vi "ADC_wave_sample.vi"() -> ()   [LabVIEW 2022 SP3]
uses:
  libdaqVI.lvlib
panel:
  in  "量程选择":T1(ring)=enum."0-5V"
  in  "AIN7":bool=TRUE
  in  "AIN5":bool=TRUE
  in  "AIN6":bool=TRUE
  in  "AIN4":bool=TRUE
  in  "AIN3":bool=TRUE
  in  "AIN2":bool=TRUE
  in  "AIN1":bool=TRUE
  in  "AIN0":bool=TRUE
  in  "wave_len":i32=1000 caption="波形显示长度"
  out "Total_len":i32 caption="每通道累计采集数据长度"
  in  "停止采集":bool
  in  "开始采集":bool
  out "设备名称":string
  in  "采样模式":enum16{"序列采样", "分组采样", "同步采样"}(ring)
  in  "组间隔(us)":u32=1000
  in  "采样次数":u32
  in  "采样频率(Hz)":u32=10000 format="%.0p"
  out "采集卡状态":bool
  out "设备数量":u32
  out "波形图":dbl[][](graph)
  in  "退出程序":bool
  # "范例说明：\n1、范例支持的采集卡：DAQ-USB3212、DAQ-USB3213、DAQ-USB3214\n2、参数配置\n1）量程选择：\nDAQ-USB3212 支持量程:0-5V\nDAQ-USB3213 支持量程:0-2.5V/0-5V/0-10V\nDAQ-USB3214 支持量程:0-2.5V/0-5V/0-10V/±2.5V/±5V/±10V\n必须选择正确的量程，否则程序会报错\n2）采样频率最大支持100kHz，同步采样时，8通道最大为10KHz\n3）采样次数，0代表无限次采样，非0值代表每通道的采样点个数\n各种采样模式之间的区别，以及详细的使用方法，请参考API手册\n3、配置正确参数之后，再开始运行程序，程序运行之后将无法修改参数\n4、程序运行之后，点击“开始采集”，进行数据采集，停止采集之后点击“开始采集”可以再次开启采集过程；"
  # "DAQ-ADC1波形采样演示程序"
  # "通道选择"
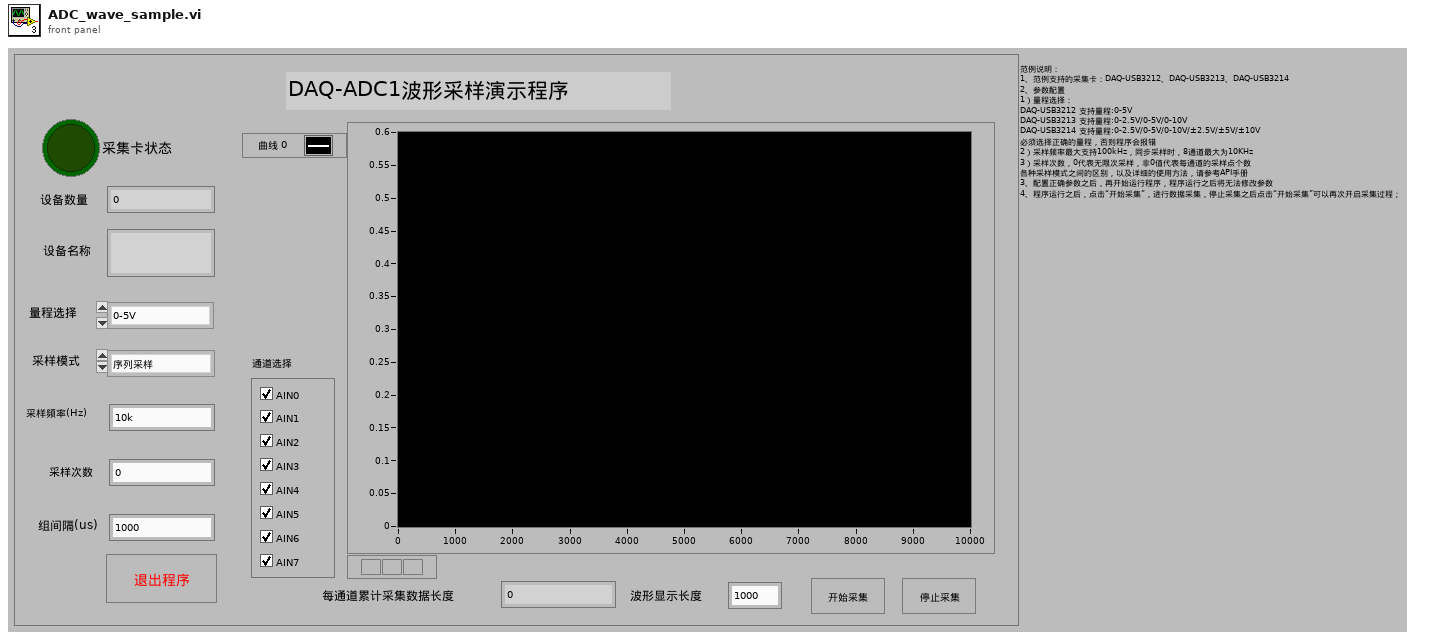
[diagram p1: front panel]
types:
  T1 = enum16{"0-1V", "0-2V", "0-2.5V", "0-5V", "0-10V", "±78.125mV", "±156.25mV", "±312.5mV", "±0.256V", "±0.512V", "±0.625V", "±1V", "±1.024V", "±1.25V", "±2V", "±2.048V", "±2.5V", "±4.096V", "±5.0V", "±10V", "0-20mA", "±20mA", "0-40mA", "±40mA"}
  T2 = cluster{"channel_list ":u8[], "channel_count":u8, "sample_mode":u8, "frequency":u32, "cycles":u32, "group_interval":u32}
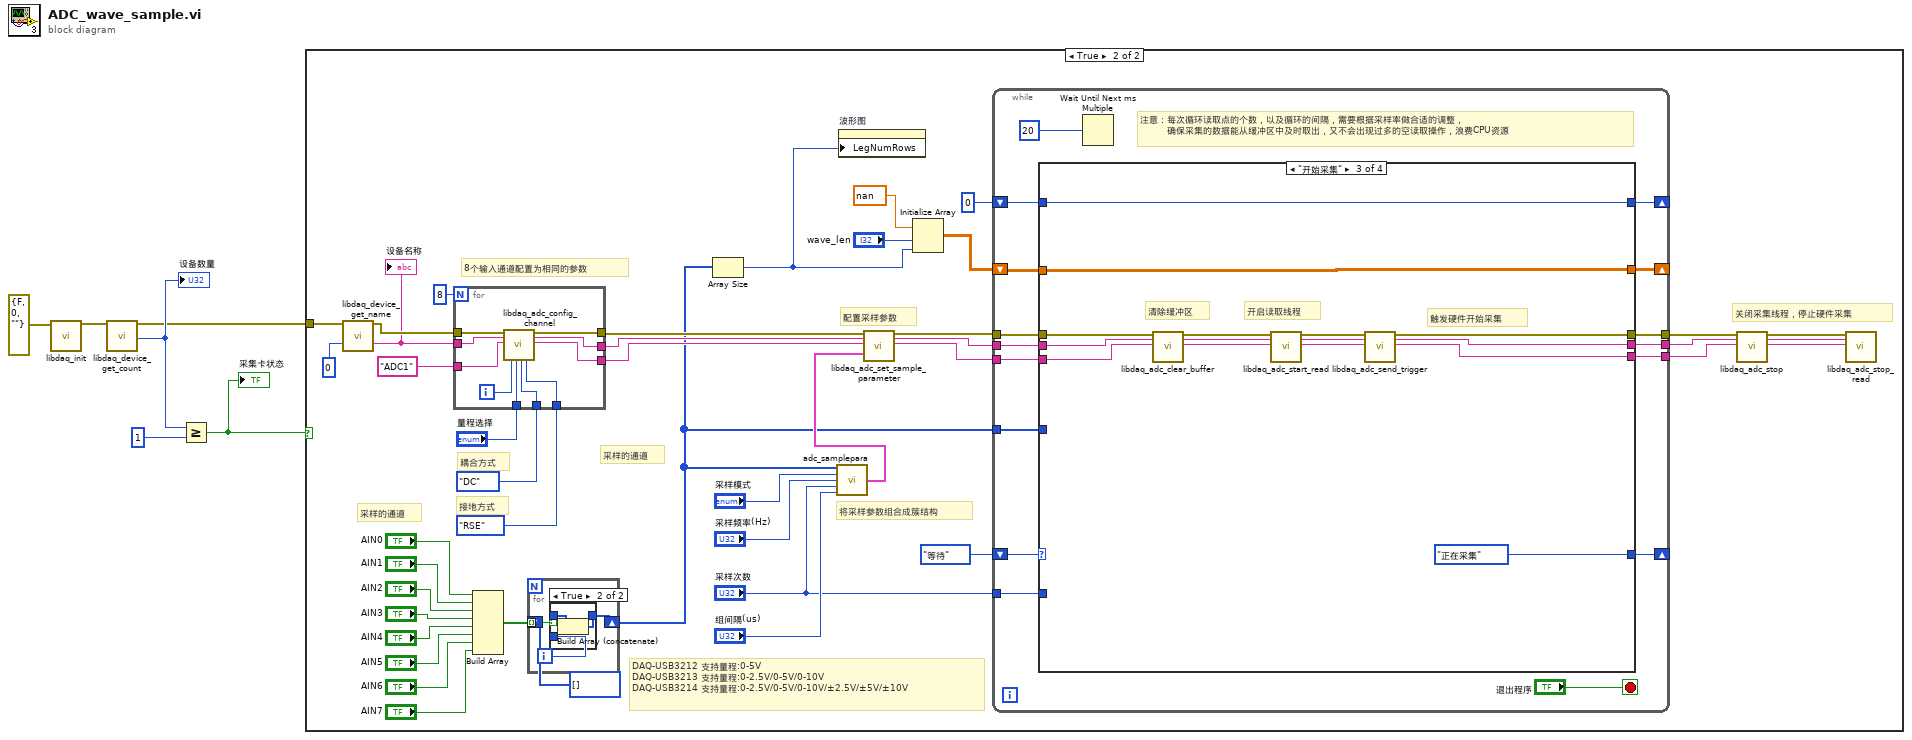
[diagram p0: block diagram]
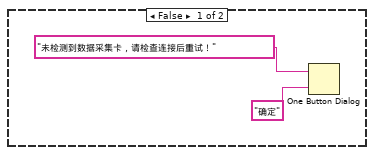
[diagram p2: hidden frame]
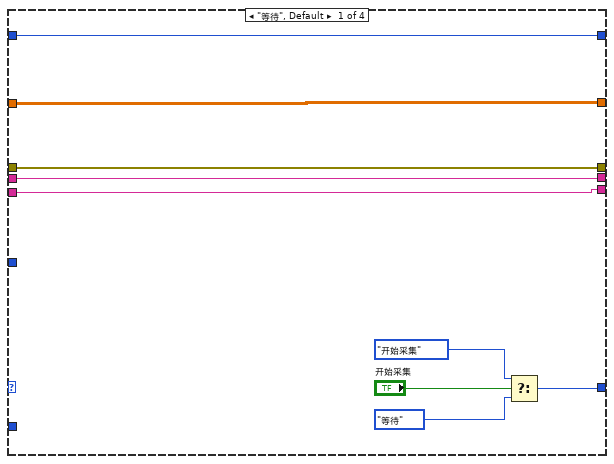
[diagram p4: hidden frame]
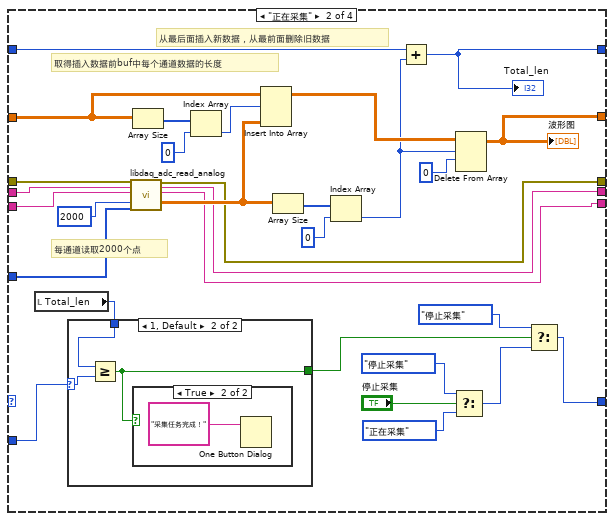
[diagram p5: hidden frame]
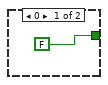
[diagram p6: hidden frame]
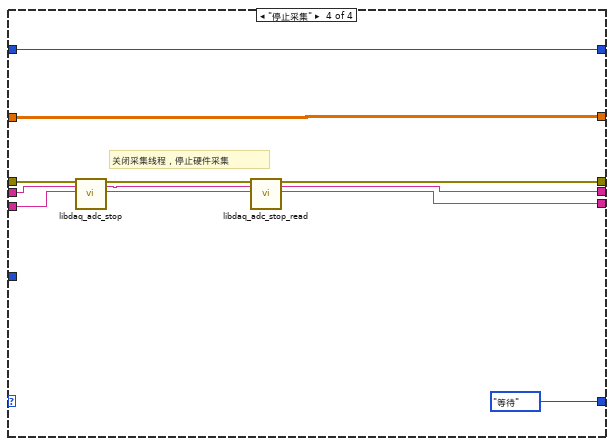
[diagram p8: hidden frame]
diagram:
  n1 = call "libdaq_init.vi"("error in (no error)"=errorcluster {"status"=FALSE, "code"=0, "source"=""}) -> ("error out"=w4:errorcluster)  [unwired: 18 in]
  n2 = call "libdaq_device_get_count.vi"("error in (no error)"=w4) -> ("error out"=w1:errorcluster, "device_count"=w2:i32)  [unwired: 17 in]
  "设备数量" <- w2
  n3 = Greater Or Equal?(x=w2, y=u32 1 ("name length")) -> (x >= y?=w3:bool)
  "采集卡状态" <- w3
  n4 = case shown="True" w3 {
    tunnel: w1 -> [_ w51]
    frame False {
      n5 = One Button Dialog(message="未检测到数据采集卡，请检查连接后重试！" ("消息"), button name ("OK")="确定" ("按钮名称（“确定”）")) -> ()  [unwired: 1 out]
    }
    frame True {
      # "关闭采集线程，停止硬件采集"
      # "采样的通道"
      # "DAQ-USB3212 支持量程:0-5V\nDAQ-USB3213 支持量程:0-2.5V/0-5V/0-10V\nDAQ-USB3214 支持量程:0-2.5V/0-5V/0-10V/±2.5V/±5V/±10V"
      # "采样的通道"
      # "接地方式"
      # "耦合方式"
      # "将采样参数组合成簇结构"
      # "配置采样参数"
      # "8个输入通道配置为相同的参数"
      n6 = call "libdaq_device_get_name.vi"("error in (no error)"=w51, "device_index"=u32 0 ("name length")) -> ("error out"=w50:errorcluster, "device_name"=w38:string)  [unwired: 16 in]
      "设备名称" <- w38
      n7 = for {
        N: 8 -> [_]
        tunnel: w50 -> [w69]
        tunnel: [w68] -> w46
        tunnel: [w64] -> w42
        tunnel: [w63] -> w41
        tunnel: "ADC1" ("module_name") -> [w65]
        tunnel: enum8{"DC", "AC"}."DC" ("couplemode") -> [w67]
        tunnel: enum8{"RSE", "NRSE", "DIFF"}."RSE" ("refground") -> [w66]
        tunnel: w38 -> [w61]
        tunnel: "量程选择" -> [w60]
        i -> [w62]
        n8 = call "libdaq_adc_config_channel.vi"("error in (no error)"=w69, "device_name"=w61, "module_name"=w65, "channel"=w62, "range"=w60, "couplemode"=w67, "refground"=w66) -> ("error out"=w68:errorcluster, "device_name"=w64:string, "module_name"=w63:string)  [unwired: 10 in]
      }
      n9 = Build Array("AIN0", "AIN1", "AIN2", "AIN3", "AIN4", "AIN5", "AIN6", "AIN7") -> (w19:bool[])
      n10 = for {
        tunnel: w19 -> [w55] mode=indexing
        shift-right: [w52] -> w18
        shift-left: i32[] [] ("数组") -> [w53]
        i -> [w54]
        n11 = case shown="True" w55 {
          tunnel: w53 -> [w56 w58]
          tunnel: w54 -> [_ w57]
          tunnel: [w56 w59] -> w52
          frame False {
          }
          frame True {
            n12 = Build Array (concatenate)(w58, w57) -> (w59:i32[])
          }
        }
      }
      n13 = Array Size(array=w18) -> (size(s)=w17:i32)
      n14 = call "adc_samplepara.vi"("channel_list"=w18, "sample_mode"="采样模式", "frequency"="采样频率(Hz)", "cycles"="采样次数", "group_interval"="组间隔(us)") -> ("adc_samplepara"=w40:T2)  [unwired: 10 in]
      n15 = property on="波形图" class="WFGraph (strict)"("LegNumRows"=w17) -> ()  [unwired: 2 in, 2 out]
      n16 = call "libdaq_adc_set_sample_parameter.vi"("error in (no error)"=w46, "device_name"=w42, "module_name"=w41, "adc_samplepara"=w40) -> ("error out"=w35:errorcluster, "device_name"=w33:string, "module_name"=w34:string)  [unwired: 13 in]
      n17 = Initialize Array(nan ("元素"), "wave_len", w17) -> (w29:dbl[][])
      n18 = while {
        tunnel: w35 -> [w85]
        tunnel: w33 -> [w84]
        tunnel: w34 -> [w83]
        shift-right: [w82] -> _
        shift-left: w29 -> [w73]
        tunnel: w18 -> [w81]
        shift-right: [w78] -> _
        shift-left: enum16{"停止采集", "开始采集", "正在采集", "等待"}."等待" -> [w79]
        tunnel: "采样次数" -> [w76]
        shift-right: [w74] -> _
        shift-left: 0 ("维数大小") -> [w75]
        tunnel: [w72] -> w12
        tunnel: [w71] -> w11
        tunnel: [w70] -> w10
        stop <- "退出程序" stop-if-true
        # "注意：每次循环读取点的个数，以及循环的间隔，需要根据采样率做合适的调整，\n         确保采集的数据能从缓冲区中及时取出，又不会出现过多的空读取操作，浪费CPU资源"
        n19 = case shown="\"开始采集\"" w79 {
          tunnel: w85 -> [w88 w124 w143 w153]
          tunnel: w84 -> [w87 w123 w142 w152]
          tunnel: w83 -> [w86 w122 w141 w151]
          tunnel: [w94 w108 w135 w155] -> w82
          tunnel: w81 -> [_ w120 _ _]
          tunnel: [w93 w114 enum16{"停止采集", "开始采集", "正在采集", "等待"}."正在采集" enum16{"停止采集", "开始采集", "正在采集", "等待"}."等待"] -> w78
          tunnel: w76 -> [_ w117 _ _]
          tunnel: w75 -> [w89 w107 w133 w154]
          tunnel: [w89 w106 w133 w154] -> w74
          tunnel: w73 -> [w94 w104 w135 w155]
          tunnel: [w88 w97 w132 w147] -> w72
          tunnel: [w87 w96 w131 w146] -> w71
          tunnel: [w86 w95 w130 w145] -> w70
          frame "等待", Default {
            n20 = Select(t=enum16{"停止采集", "开始采集", "正在采集", "等待"}."开始采集", s="开始采集", f=enum16{"停止采集", "开始采集", "正在采集", "等待"}."等待") -> (s? t:f=w93:enum16{"停止采集", "开始采集", "正在采集", "等待"})
          }
          frame "正在采集" {
            # "取得插入数据前buf中每个通道数据的长度"
            # "从最后面插入新数据，从最前面删除旧数据"
            # "每通道读取2000个点"
            n21 = local read "Total_len"() -> (w105:i32)
            n22 = case shown="1, Default" w117 {
              selector: w117 -> [_ w128]
              tunnel: [FALSE w127] -> w116
              tunnel: w105 -> [_ w126]
              frame 0 {
              }
              frame 1, Default {
                n23 = Greater Or Equal?(x=w126, y=w128) -> (x >= y?=w127:bool)
                n24 = case shown="True" w127 {
                  frame False {
                  }
                  frame True {
                    n25 = One Button Dialog(message="采集任务完成！" ("消息")) -> ()  [unwired: 1 in, 1 out]
                  }
                }
              }
            }
            n26 = call "libdaq_adc_read_analog.vi"("error in (no error)"=w124, "device_name"=w123, "module_name"=w122, "datalen_ch"=u32 2000 ("milliseconds to wait"), "channel_list"=w120) -> ("error out"=w97:errorcluster, "device_name"=w96:string, "module_name"=w95:string, "databuf"=w100:dbl[][])  [unwired: 11 in]
            n27 = Array Size(array=w104) -> (size(s)=w111:i32[])
            n28 = Index Array(array=w111, index=0 ("索引")) -> (element=w103:i32)
            n29 = Insert Into Array(array=w104, index (row)=w103, new element=w100) -> (w109:dbl[][])  [unwired: 1 in]
            n30 = Array Size(array=w100) -> (size(s)=w101:i32[])
            n31 = Index Array(array=w101, index=0 ("索引")) -> (element=w99:i32)
            n32 = Add(x=w107, y=w99) -> (x+y=w106:i32)
            "Total_len" <- w106
            n33 = Select(t=enum16{"停止采集", "开始采集", "正在采集", "等待"}."停止采集", s="停止采集", f=enum16{"停止采集", "开始采集", "正在采集", "等待"}."正在采集") -> (s? t:f=w113:enum16{"停止采集", "开始采集", "正在采集", "等待"})
            n34 = Delete From Array(array=w109, length=w99, index (row)=0 ("索引 (行)")) -> (array with subset deleted=w108:dbl[][])  [unwired: 1 in, 1 out]
            "波形图" <- w108
            n35 = Select(t=enum16{"停止采集", "开始采集", "正在采集", "等待"}."停止采集", s=w116, f=w113) -> (s? t:f=w114:enum16{"停止采集", "开始采集", "正在采集", "等待"})
          }
          frame "开始采集" {
            # "触发硬件开始采集"
            # "开启读取线程"
            # "清除缓冲区"
            n36 = call "libdaq_adc_clear_buffer.vi"("error in (no error)"=w143, "device_name"=w142, "module_name"=w141) -> ("error out"=w139:errorcluster, "device_name"=w138:string, "module_name"=w140:string)  [unwired: 14 in]
            n37 = call "libdaq_adc_start_read.vi"("error in (no error)"=w139, "device_name"=w138, "module_name"=w140) -> ("error out"=w137:errorcluster, "device_name"=w134:string, "module_name"=w136:string)  [unwired: 14 in]
            n38 = call "libdaq_adc_send_trigger.vi"("error in (no error)"=w137, "device_name"=w134, "module_name"=w136) -> ("error out"=w132:errorcluster, "device_name"=w131:string, "module_name"=w130:string)  [unwired: 14 in]
          }
          frame "停止采集" {
            # "关闭采集线程，停止硬件采集"
            n39 = call "libdaq_adc_stop.vi"("error in (no error)"=w153, "device_name"=w152, "module_name"=w151) -> ("error out"=w150:errorcluster, "device_name"=w149:string, "module_name"=w148:string)  [unwired: 14 in]
            n40 = call "libdaq_adc_stop_read.vi"("error in (no error)"=w150, "device_name"=w149, "module_name"=w148) -> ("error out"=w147:errorcluster, "device_name"=w146:string, "module_name"=w145:string)  [unwired: 14 in]
          }
        }
        n41 = Wait Until Next ms Multiple(millisecond multiple=u32 20 ("milliseconds to wait")) -> ()  [unwired: 1 out]
      }
      n42 = call "libdaq_adc_stop.vi"("error in (no error)"=w12, "device_name"=w11, "module_name"=w10) -> ("error out"=w15:errorcluster, "device_name"=w14:string, "module_name"=w13:string)  [unwired: 14 in]
      n43 = call "libdaq_adc_stop_read.vi"("error in (no error)"=w15, "device_name"=w14, "module_name"=w13) -> ()  [unwired: 14 in, 3 out]
    }
  }
